vi "Sensor Mesurament from phone and hercules.vi"() -> ()   [LabVIEW 2012]
uses:
  <vilib>/Instr/_visa.llb/VISA Configure Serial Port (Instr).vi
  <vilib>/Utility/file.llb/Write To Spreadsheet File (DBL).vi
  <vilib>/Utility/file.llb/Read From Spreadsheet File (DBL).vi
  <vilib>/Utility/file.llb/Write To Spreadsheet File (string).vi
  <vilib>/Utility/file.llb/Read From Spreadsheet File (string).vi
  <vilib>/Analysis/NI_AALBase.lvlib
panel:
  out "Control Option":string
  out "Dati":dbl[][](array[numeric])
  in  "Tab Control":T1(tab)
  out "?":bool
  in  "QUIT":bool
  out "Off/On":bool
  in  "Unit":u32(ring)=1000 items=["hr"=3600000, "min"=60000, "sec"=1000, "ms"=1]
  in  "Timer":bool
  in  "Magnitude":bool
  in  "Filter":u16
  in  "?":bool
  in  "?":bool
  in  "?":bool
  in  "?":bool
  in  "?":bool
  in  "?":bool
  in  "?":bool
  in  "?":bool
  in  "?":bool
  in  "?":bool
  in  "?":bool
  in  "?":bool
  in  "?":bool
  in  "?":bool
  in  "read bluetooth":bool
  in  "VISA resource name":refnum<visa-resource-name>="COM4"
  out "Bytes at Port":u32
  in  "baud rate (9600)":u32=9600
  in  "stop and Save":bool
  out "dati ist":dbl[](array[numeric])
  out "?":waveform(dbl)[](graph)
  in  "dt":dbl=100.0
  in  "Save path":path=path "C:/Users/leona/Desktop/progetto misure/File/Saves"
  out "start data/time":string
  out "stop data/time":string
  out "Max":dbl[](array[numeric])
  out "Min":dbl[](array[numeric])
  out "Mean":dbl[](array[numeric])
  out "St. dev":dbl[](array[numeric])
  out "Variance":dbl[](array[numeric])
  in  "data bits (8)":u16=8 min=5 max=8 step=1
  in  "parity (0:none)":enum16{"None", "Odd", "Even", "Mark", "Space"}(ring)
  in  "stop bits (10: 1 bit)":u16(ring)=10 items=["1.0"=10, "1.5"=15, "2.0"=20]
  in  "flow control (0:none)":u16(ring) items=["None", "XON/XOFF", "RTS/CTS", "XON/XOFF & RTS/CTS", "DTR/DSR", "XON/XOFF & DTR/DSR"]
  out "Tick count":u32
  in  "Timer":dbl
  in  "Both":bool
  in  "?":bool
  in  "?":bool
  in  "?":bool
  in  "?":bool
  in  "?":bool
  in  "?":bool
  in  "?":bool
  in  "?":bool
  in  "?":bool
  in  "?":bool
  in  "?":bool
  in  "?":bool
  in  "?":bool
  in  "?":bool
  in  "file 1":path
  out "Max 1":dbl[](array[numeric])
  out "Min 1":dbl[](array[numeric])
  out "Mean 1":dbl[](array[numeric])
  out "St. Dev 1":dbl[](array[numeric])
  out "Varian 1":dbl[](array[numeric])
  in  "dt 1":dbl=100.0
  in  "Filter 1":u16
  out "?":waveform(dbl)[](graph)
  out "Varian 2":dbl[](array[numeric])
  out "St. Dev 2":dbl[](array[numeric])
  out "Mean 2":dbl[](array[numeric])
  out "Min 2":dbl[](array[numeric])
  out "Max 2":dbl[](array[numeric])
  in  "file 2":path
  in  "Filter 2":u16
  in  "dt 2":dbl=100.0
  out "Start data 2":string
  out "Stop data 2":string
  out "Start data 1":string
  out "Stop data 1":string
  out "?":waveform(dbl)[](graph)
  in  "Stop Load":bool
  in  "Load":bool
  in  "Filter both":u16
  in  "dt both":dbl=100.0
  out "Dati 1":dbl[][](array[numeric])
  out "Dati 2":dbl[][](array[numeric])
  out "Delta T 1(s)":dbl
  out "Delta T2 (s)":dbl
  in  "?":bool
  in  "?":bool
  in  "?":bool
  in  "?":bool
  in  "?":bool
  in  "?":bool
  in  "?":bool
  in  "?":bool
  in  "?":bool
  in  "?":bool
  in  "?":bool
  in  "?":bool
  in  "?":bool
  in  "?":bool
  out "Waveform Graph":waveform(dbl)[](graph)
  out "?":dbl[][](array[numeric])
  in  "file path":path=path "C:/Users/leona/Desktop/progetto misure/Telefono_COM4/Dati_Telefono_deltaT.log"
  in  "Read file":bool
  out "Max 3":dbl[](array[numeric])
  out "Min 3":dbl[](array[numeric])
  out "Mean 3":dbl[](array[numeric])
  out "St. dev 3":dbl[](array[numeric])
  out "Variance 3":dbl[](array[numeric])
  in  "stop":bool
  in  "Filter 3":u16
  in  "dt 3":dbl=100.0
  out "Stato DIst (disabilitato)":bool
  in  "Lock Distance":bool
  out "Load File":bool
  out "Read Bluetooth":bool
  out "Read File":bool
  out "Admin":bool
  out "Stato locat (disabilitato)":bool
  in  "Lock Location":bool
  in  "Add":bool
  in  "PASS":string
  in  "ID":string
  in  "Show":bool
  out "Username & Password":string[][](array[string])
  in  "Delete":bool
  in  "Delete ID":string
  out "Result":string
  # "You have successfully logged in!"
  # "Read Bluetooth: read data from your phone sensors"
  # "Load file: Let you load old file"
  # "Read File: read data from Hercules software"
  # "Admin option: Admin exclusive options"
  # "xxxxxxxxxxxxxxxxxxxxxxxxxxxxxxxxxxxxx\n\n                       Sensor Project\n\nxxxxxxxxxxxxxxxxxxxxxxxxxxxxxxxxxxxxx"
  # "Acc X"
  # "Acc Y"
  # "Acc Z"
  # "Velo X"
  # "Velo Y"
  # "Velo Z"
  # "Azimuth"
  # "Pitch"
  # "Roll"
  # "Distance"
  # "Lat"
  # "Lon"
  # "Altitude"
  # "Speed"
  # "Connection option"
  # "Timer option"
  # "off/on"
  # "Acc X"
  # "Acc Y"
  # "Acc Z"
  # "Velo X"
  # "Velo Y"
  # "Velo Z"
  # "Azimuth"
  # "Pitch"
  # "Roll"
  # "Distance"
  # "Lat"
  # "Lon"
  # "Altitude"
  # "Speed"
  # "Acc X"
  # "Acc Y"
  # "Acc Z"
  # "Velo X"
  # "Velo Y"
  # "Velo Z"
  # "Azimuth"
  # "Pitch"
  # "Roll"
  # "Distance"
  # "Lat"
  # "Lon"
  # "Altitude"
  # "Speed"
  # "Login option"
  # "Lock option"
  # "Active functions"
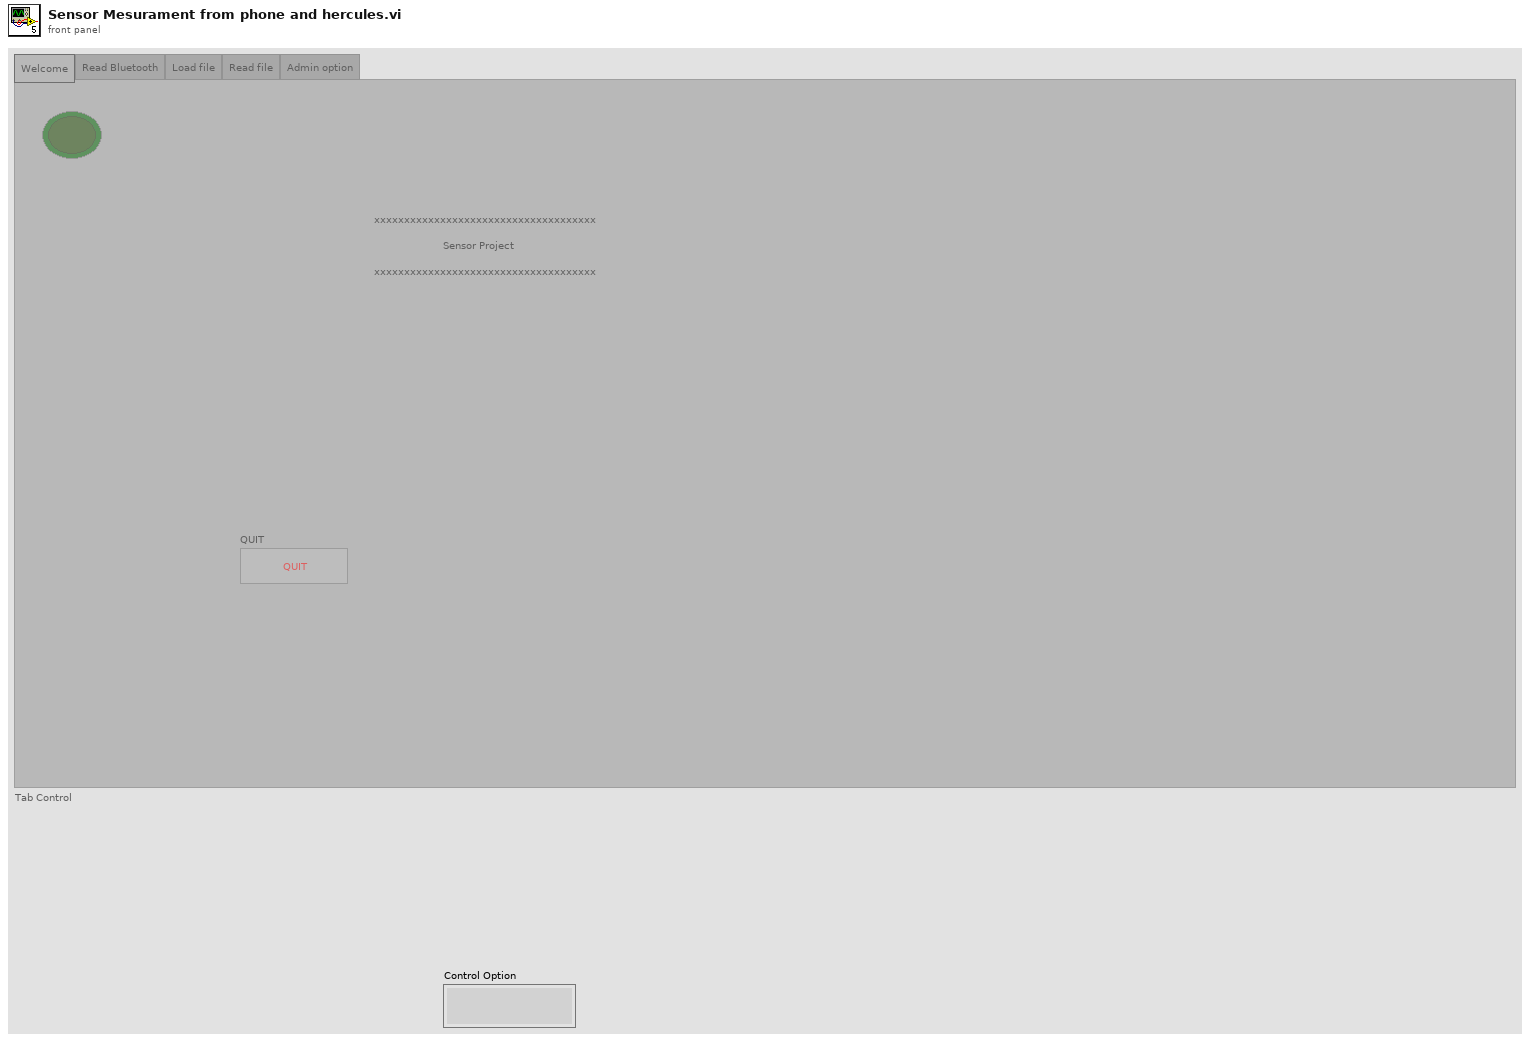
[diagram p1: front panel]
types:
  T1 = enum32{"Welcome", "Read Bluetooth", "Load file", "Read file", "Admin option"}
  T2 = enum8{"Enabled", "Disabled", "Disabled and Grayed Out"}
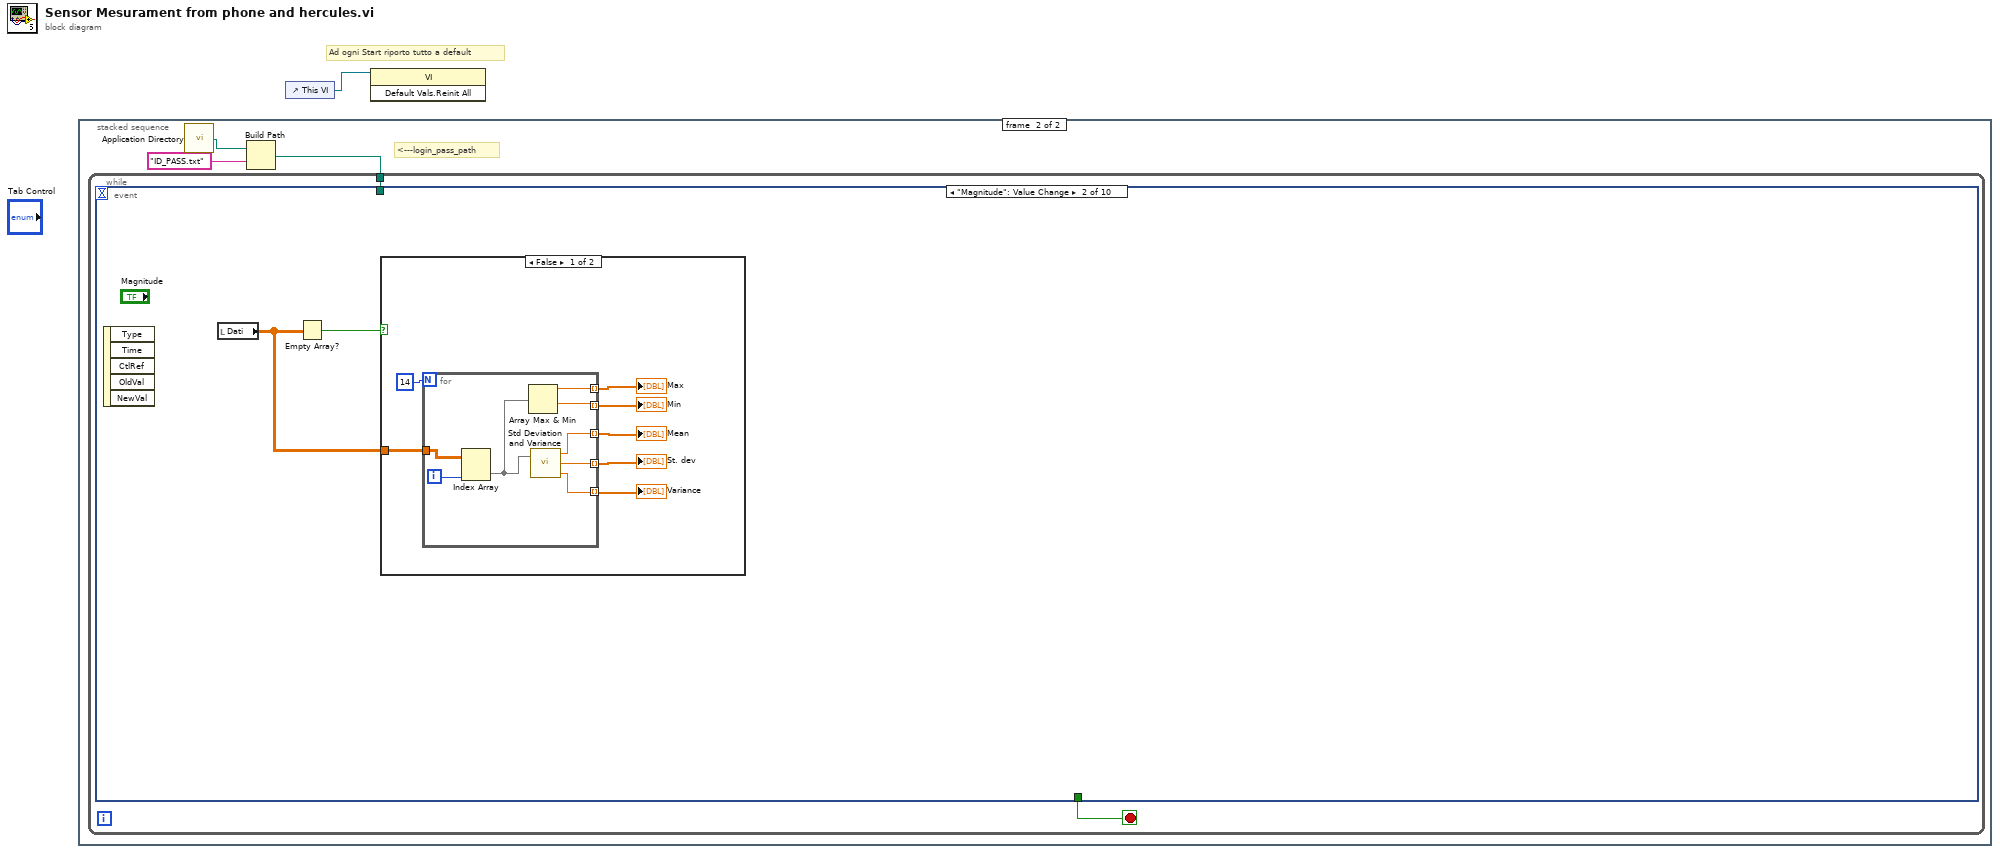
[diagram p0: block diagram]
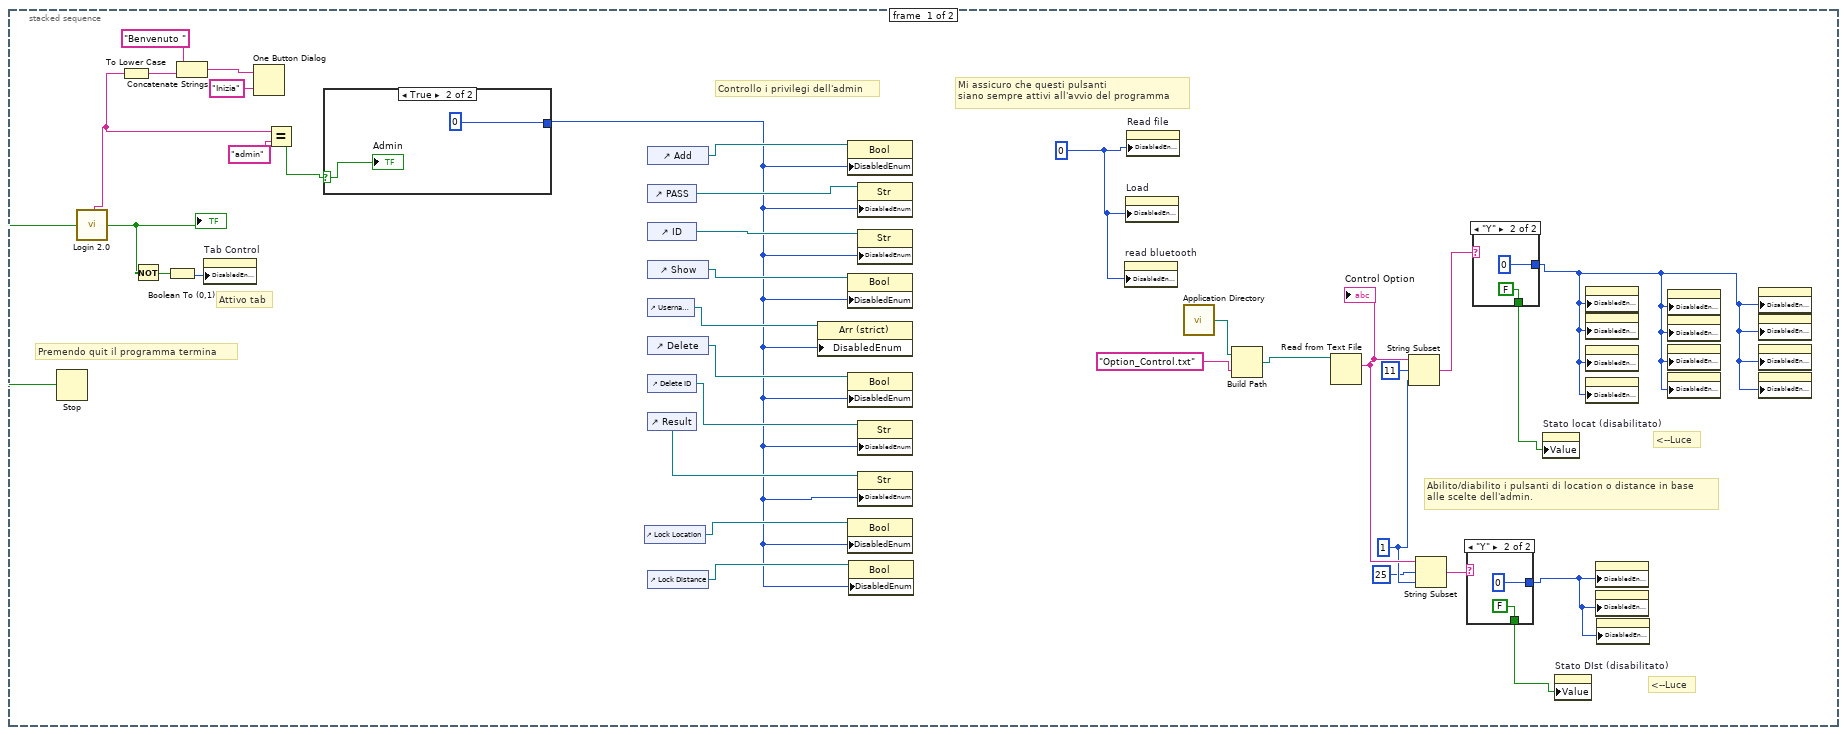
[diagram p2: hidden frame]
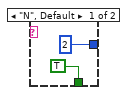
[diagram p3: hidden frame]
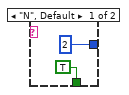
[diagram p4: hidden frame]
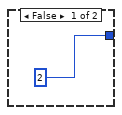
[diagram p5: hidden frame]
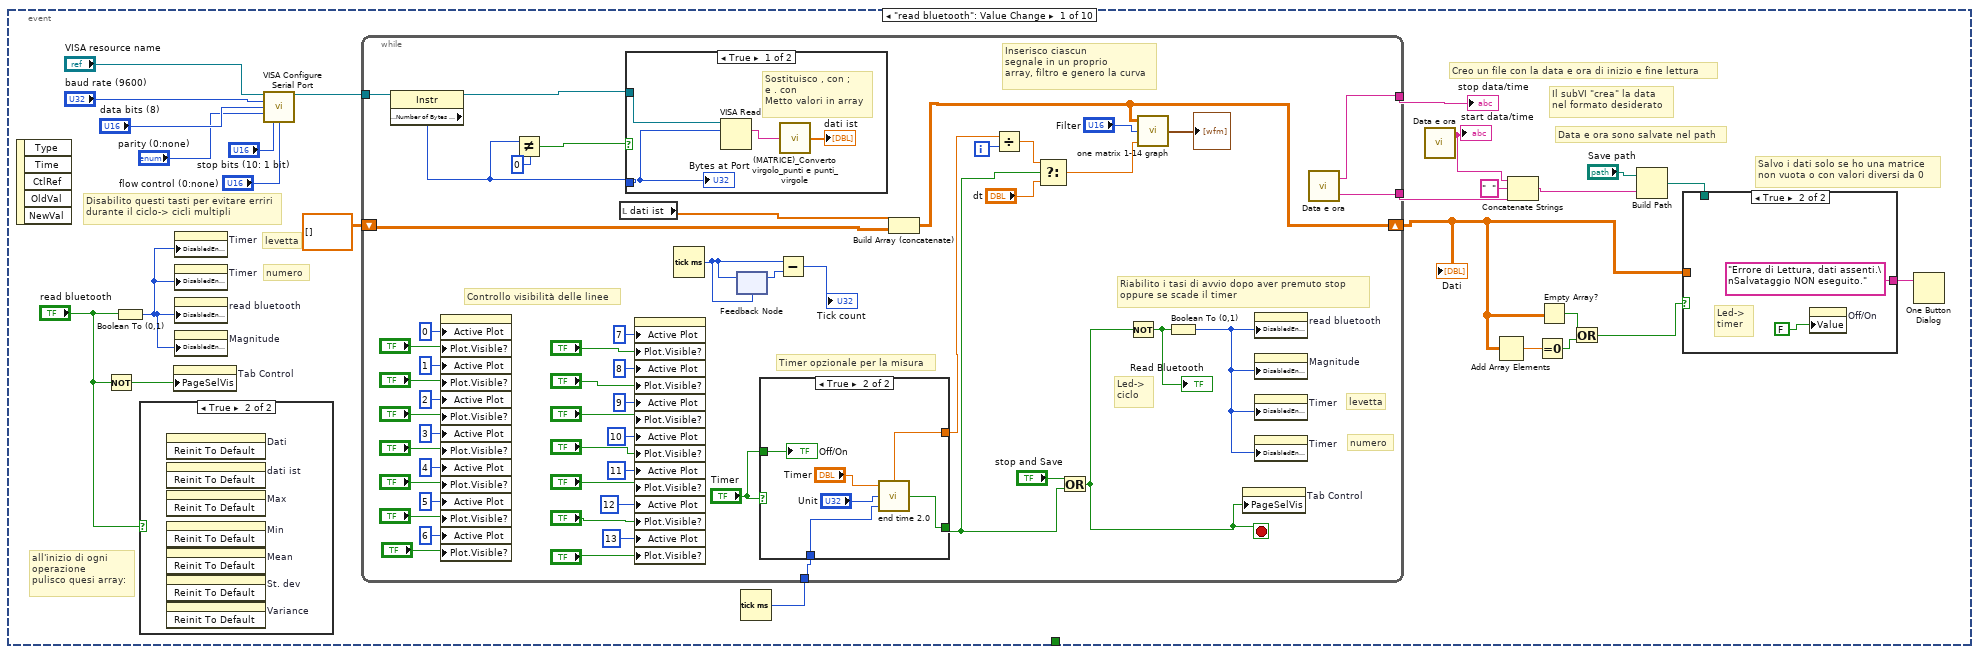
[diagram p6: hidden frame]
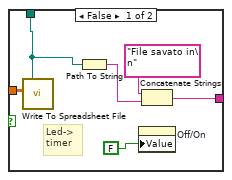
[diagram p8: hidden frame]
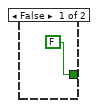
[diagram p9: hidden frame]
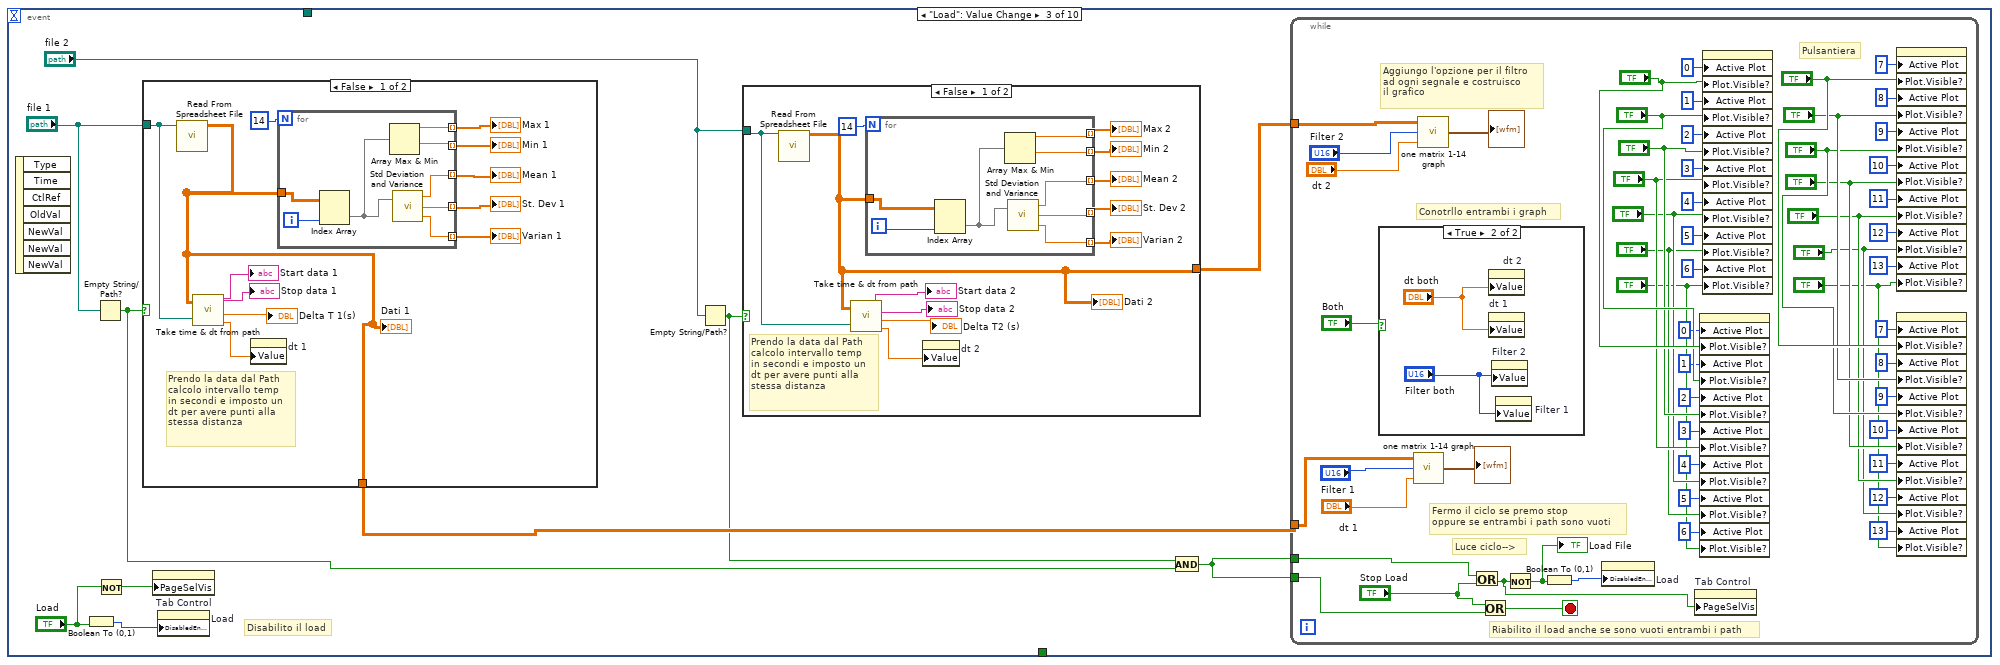
[diagram p12: hidden frame]
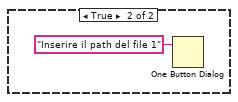
[diagram p14: hidden frame]
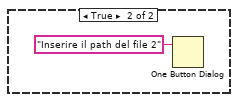
[diagram p15: hidden frame]
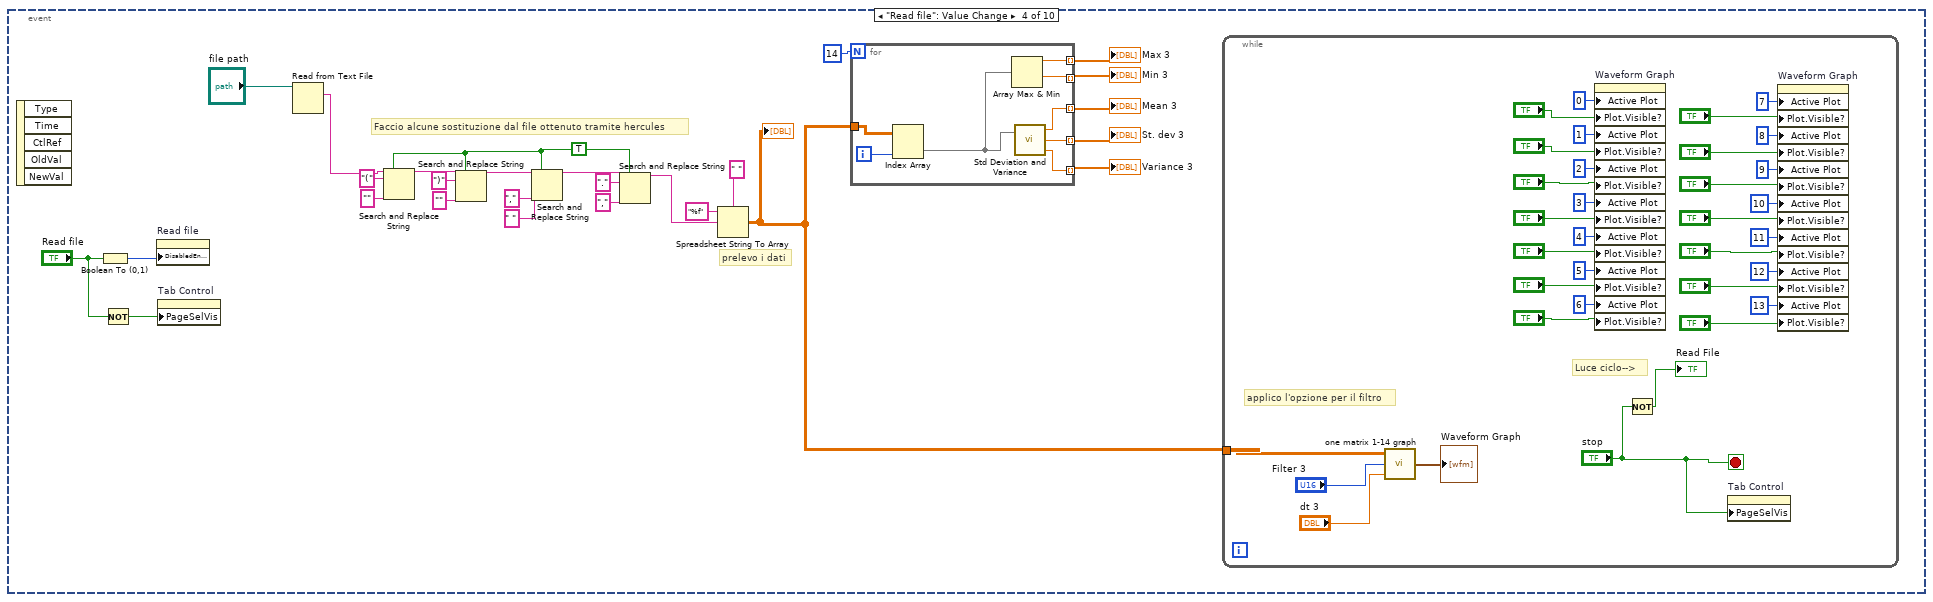
[diagram p16: hidden frame]
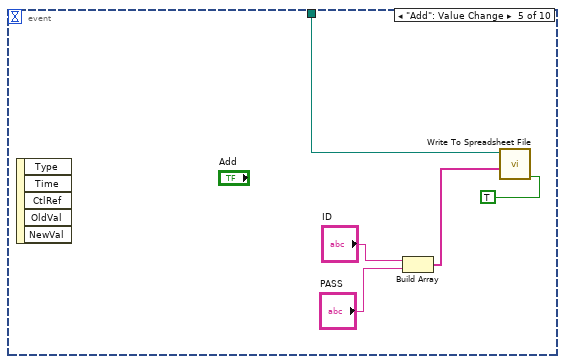
[diagram p17: hidden frame]
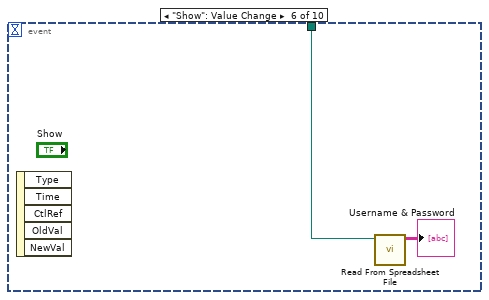
[diagram p18: hidden frame]
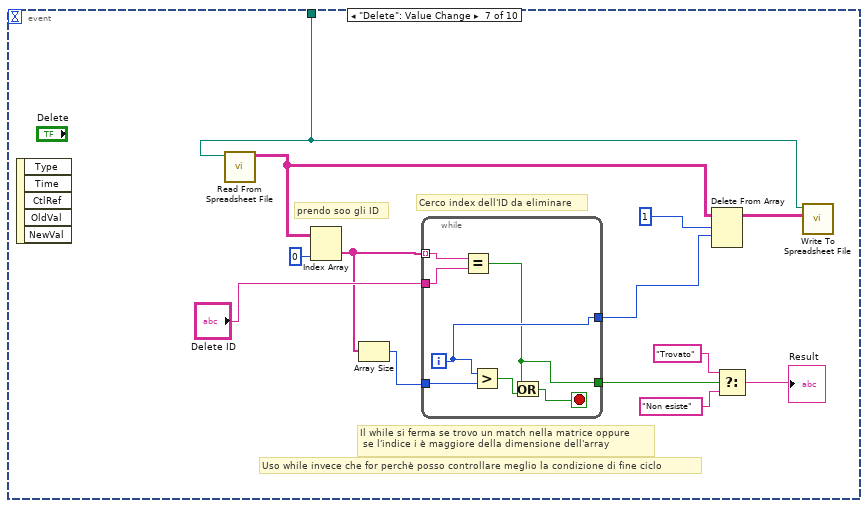
[diagram p19: hidden frame]
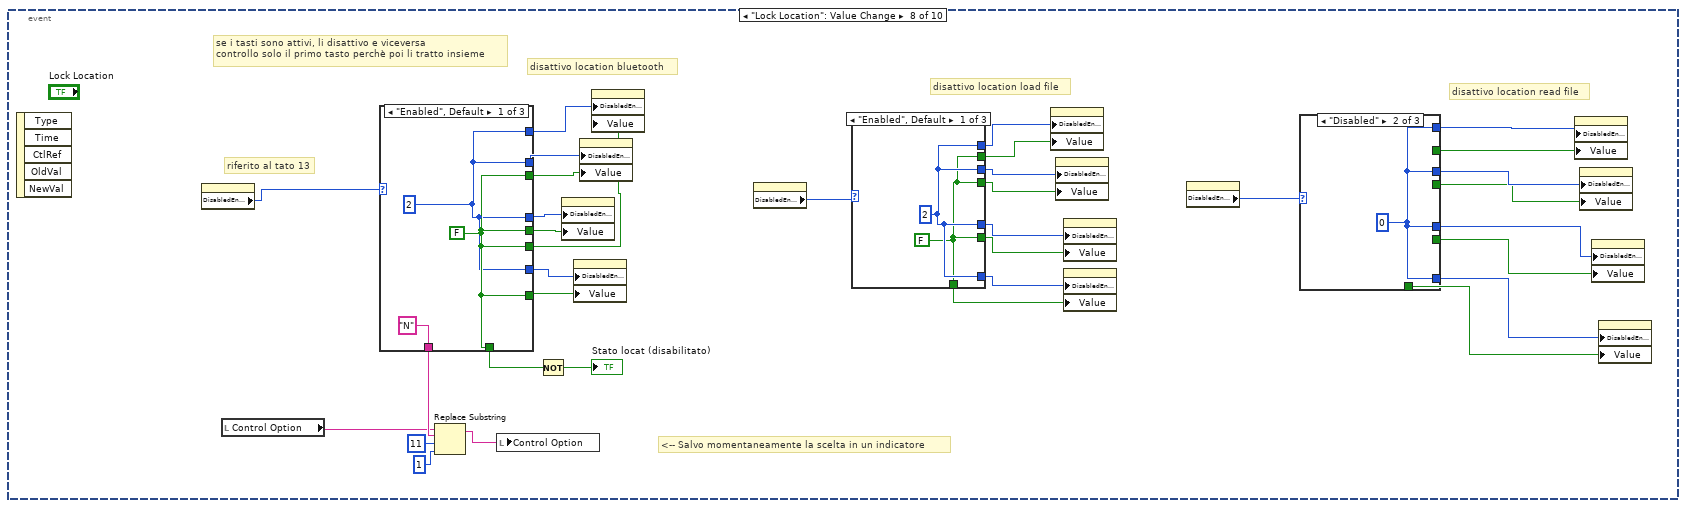
[diagram p20: hidden frame]
diagram:
  # "Ad ogni Start riporto tutto a default"
  n1 = stacked-sequence {
    frame #0 {
      w12 = 1 ("length (rest)")
      w28 = 0
      # "<--Luce"
      # "<--Luce"
      # "Abilito/diabilito i pulsanti di location o distance in base\nalle scelte dell'admin."
      # "Premendo quit il programma termina"
      # "Attivo tab"
      # "Controllo i privilegi dell'admin"
      # "Mi assicuro che questi pulsanti\nsiano sempre attivi all'avvio del programma"
      n2 = call "Login 2.0.vi"() -> ("quit led"=w15:bool, "UTENTE"=w17:string, 2:w16:bool)
      "?" <- w16
      n3 = Stop(stop? (T)=w15) -> ()
      n4 = To Lower Case(string=w17) -> (all lower case string=w21:string)
      n5 = Not(x=w16) -> (.not. x?=w18:bool)
      n6 = Boolean To (0,1)(Boolean=w18) -> (0, 1=w27:i16)
      n7 = Concatenate Strings("Benvenuto " ("string"), w21) -> (w23:string)
      n8 = property on="Tab Control" class="TabCtl (strict)"("DisabledEnum"=w27) -> ()  [unwired: 2 in, 2 out]
      n9 = One Button Dialog(message=w23, button name ("OK")="Inizia") -> ()  [unwired: 1 out]
      n10 = Equal?(x=w17, y="admin") -> (x = y?=w26:bool)
      n11 = case shown="True" w26 {
        selector: w26 -> [_ w47]
        tunnel: [2 0] -> w19
        frame False {
        }
        frame True {
          "Admin" <- w47
        }
      }
      n12 = control-ref of="Lock Location"() -> (w25:refnum<vi>)
      n13 = control-ref of="Add"() -> (w36:refnum<vi>)
      n14 = control-ref of="PASS"() -> (w35:refnum<vi>)
      n15 = control-ref of="ID"() -> (w34:refnum<vi>)
      n16 = control-ref of="Show"() -> (w33:refnum<vi>)
      n17 = control-ref of="Username & Password"() -> (w32:refnum<vi>)
      n18 = control-ref of="Delete"() -> (w31:refnum<vi>)
      n19 = control-ref of="Delete ID"() -> (w30:refnum<vi>)
      n20 = control-ref of="Result"() -> (w29:refnum<vi>)
      n21 = control-ref of="Lock Distance"() -> (w20:refnum<vi>)
      n22 = property class="Arr (strict)"(reference=w32, "DisabledEnum"=w19) -> ()  [unwired: 1 in, 2 out]
      n23 = property class="Bool"(reference=w36, "DisabledEnum"=w19) -> ()  [unwired: 1 in, 2 out]
      n24 = property class="Bool"(reference=w33, "DisabledEnum"=w19) -> ()  [unwired: 1 in, 2 out]
      n25 = property class="Bool"(reference=w31, "DisabledEnum"=w19) -> ()  [unwired: 1 in, 2 out]
      n26 = property class="Bool"(reference=w25, "DisabledEnum"=w19) -> ()  [unwired: 1 in, 2 out]
      n27 = property class="Bool"(reference=w20, "DisabledEnum"=w19) -> ()  [unwired: 1 in, 2 out]
      n28 = property class="Str"(reference=w35, "DisabledEnum"=w19) -> ()  [unwired: 1 in, 2 out]
      n29 = property class="Str"(reference=w34, "DisabledEnum"=w19) -> ()  [unwired: 1 in, 2 out]
      n30 = property class="Str"(reference=w30, "DisabledEnum"=w19) -> ()  [unwired: 1 in, 2 out]
      n31 = property class="Str"(reference=w29, "DisabledEnum"=w19) -> ()  [unwired: 1 in, 2 out]
      n32 = property on="read bluetooth" class="Bool"("DisabledEnum"=w28) -> ()  [unwired: 2 in, 2 out]
      n33 = property on="Load" class="Bool"("DisabledEnum"=w28) -> ()  [unwired: 2 in, 2 out]
      n34 = property on="Read file" class="Bool"("DisabledEnum"=w28) -> ()  [unwired: 2 in, 2 out]
      n35 = call <vilib>:"Application Directory.vi"() -> ("Application Directory"=w4:path)
      n36 = Build Path(base path=w4, name or relative path="Option_Control.txt") -> (appended path=w2:path)
      n37 = Read from Text File(file (use dialog)=w2) -> (text=w13:string)  [unwired: 3 in, 3 out]
      "Control Option" <- w13
      n38 = String Subset(string=w13, offset (0)=11, length (rest)=w12) -> (substring=w10:string)
      n39 = String Subset(string=w13, offset (0)=25, length (rest)=w12) -> (substring=w8:string)
      n40 = case shown="\"Y\"" w8 {
        tunnel: [2 0] -> w7
        tunnel: [TRUE FALSE] -> w5
        frame "N", Default {
        }
        frame "Y" {
        }
      }
      n41 = case shown="\"Y\"" w10 {
        tunnel: [2 0] -> w9
        tunnel: [TRUE FALSE] -> w6
        frame "N", Default {
        }
        frame "Y" {
        }
      }
      n42 = property on="Stato locat (disabilitato)" class="Bool (strict)"("Value"=w6) -> ()  [unwired: 2 in, 2 out]
      n43 = property on="Stato DIst (disabilitato)" class="Bool (strict)"("Value"=w5) -> ()  [unwired: 2 in, 2 out]
      n44 = property class="Bool (strict)"("DisabledEnum"=w9) -> ()  [unwired: 2 in, 2 out]
      n45 = property class="Bool (strict)"("DisabledEnum"=w9) -> ()  [unwired: 2 in, 2 out]
      n46 = property class="Bool (strict)"("DisabledEnum"=w9) -> ()  [unwired: 2 in, 2 out]
      n47 = property class="Bool (strict)"("DisabledEnum"=w9) -> ()  [unwired: 2 in, 2 out]
      n48 = property class="Bool (strict)"("DisabledEnum"=w7) -> ()  [unwired: 2 in, 2 out]
      n49 = property class="Bool (strict)"("DisabledEnum"=w7) -> ()  [unwired: 2 in, 2 out]
      n50 = property class="Bool (strict)"("DisabledEnum"=w7) -> ()  [unwired: 2 in, 2 out]
      n51 = property class="Bool (strict)"("DisabledEnum"=w9) -> ()  [unwired: 2 in, 2 out]
      n52 = property class="Bool (strict)"("DisabledEnum"=w9) -> ()  [unwired: 2 in, 2 out]
      n53 = property class="Bool (strict)"("DisabledEnum"=w9) -> ()  [unwired: 2 in, 2 out]
      n54 = property class="Bool (strict)"("DisabledEnum"=w9) -> ()  [unwired: 2 in, 2 out]
      n55 = property class="Bool (strict)"("DisabledEnum"=w9) -> ()  [unwired: 2 in, 2 out]
      n56 = property class="Bool (strict)"("DisabledEnum"=w9) -> ()  [unwired: 2 in, 2 out]
      n57 = property class="Bool (strict)"("DisabledEnum"=w9) -> ()  [unwired: 2 in, 2 out]
      n58 = property class="Bool (strict)"("DisabledEnum"=w9) -> ()  [unwired: 2 in, 2 out]
    }
    frame #1 {
      # "<---login_pass_path"
      n59 = call <vilib>:"Application Directory.vi"() -> ("Application Directory"=w51:path)
      n60 = Build Path(base path=w51, name or relative path="ID_PASS.txt") -> (appended path=w49:path)
      n61 = while {
        tunnel: w49 -> [w53]
        stop <- w52 stop-if-true
        n62 = event shown="[1] \"Magnitude\": Value Change" {
          selector: _ -> [_ _ _ _ _ _ _ _ _ _]
          dyn-events: _ -> [_ _ _ _ _ _ _ _ _ _]
          timeout: _ -> [_ _ _ _ _ _ _ _ _ _]
          tunnel: w53 -> [_ _ _ _ w351 w356 w358 _ _ _]
          tunnel: [_ _ _ _ _ _ _ _ _ "QUIT"] -> w52
          event "read bluetooth": Value Change {
            # "numero"
            # "levetta"
            # "all'inizio di ogni \noperazione\npulisco quesi array:"
            # "Salvo i dati solo se ho una matrice\nnon vuota o con valori diversi da 0"
            # "Disabilito questi tasti per evitare erriri\ndurante il ciclo-> cicli multipli"
            # "Data e ora sono salvate nel path"
            # "Il subVI \"crea\" la data\nnel formato desiderato"
            # "Creo un file con la data e ora di inizio e fine lettura"
            n63 = event-data() -> ()  [unwired: 1 in, 5 out]
            n64 = Not(x="read bluetooth") -> (.not. x?=w57:bool)
            n65 = Boolean To (0,1)(Boolean="read bluetooth") -> (0, 1=w55:i16)
            n66 = case shown="True" "read bluetooth" {
              frame False {
              }
              frame True {
                n67 = invoke on="Dati" class="Arr (strict)" method="Reinit To Default"() -> ()  [unwired: 3 in, 3 out]
                n68 = invoke on="dati ist" class="Arr (strict)" method="Reinit To Default"() -> ()  [unwired: 3 in, 3 out]
                n69 = invoke on="Max" class="Arr (strict)" method="Reinit To Default"() -> ()  [unwired: 3 in, 3 out]
                n70 = invoke on="Min" class="Arr (strict)" method="Reinit To Default"() -> ()  [unwired: 3 in, 3 out]
                n71 = invoke on="Mean" class="Arr (strict)" method="Reinit To Default"() -> ()  [unwired: 3 in, 3 out]
                n72 = invoke on="St. dev" class="Arr (strict)" method="Reinit To Default"() -> ()  [unwired: 3 in, 3 out]
                n73 = invoke on="Variance" class="Arr (strict)" method="Reinit To Default"() -> ()  [unwired: 3 in, 3 out]
              }
            }
            n74 = property on="Tab Control" class="TabCtl (strict)"("PageSelVis"=w57) -> ()  [unwired: 2 in, 2 out]
            n75 = property on="Timer" class="DigNum (strict)"("DisabledEnum"=w55) -> ()  [unwired: 2 in, 2 out]
            n76 = property on="Timer" class="Bool (strict)"("DisabledEnum"=w55) -> ()  [unwired: 2 in, 2 out]
            n77 = property on="read bluetooth" class="Bool"("DisabledEnum"=w55) -> ()  [unwired: 2 in, 2 out]
            n78 = property on="Magnitude" class="Bool"("DisabledEnum"=w55) -> ()  [unwired: 2 in, 2 out]
            n79 = call-poly "VISA Configure Serial Port"("VISA resource name"="VISA resource name", "baud rate (9600)"="baud rate (9600)", "data bits (8)"="data bits (8)", "parity (0:none)"="parity (0:none)", "stop bits (10: 1 bit)"="stop bits (10: 1 bit)", "flow control (0:none)"="flow control (0:none)") -> ("VISA resource name out"=w78:refnum<visa-resource-name>)  [unwired: 8 in, 1 out]
            n80 = Tick Count (ms)() -> (millisecond timer value=w54:u32)
            n81 = while {
              tunnel: w78 -> [w141]
              shift-right: [w87] -> w58
              shift-left: dbl[][] [] -> [w135]
              tunnel: [w111] -> w73
              tunnel: [w110] -> w74
              tunnel: w54 -> [w102]
              i -> [w89]
              stop <- w98 stop-if-true
              # "numero"
              # "levetta"
              # "Timer opzionale per la misura"
              # "Led-> \nciclo"
              # "Riabilito i tasi di avvio dopo aver premuto stop \noppure se scade il timer"
              # "Inserisco ciascun\nsegnale in un proprio\narray, filtro e genero la curva"
              # "Controllo visibilità delle linee"
              n82 = property class="Instr"(reference=w141) -> (reference out=w140:refnum<visa-resource-name>, "Serial Settings:Number of Bytes at Serial Port"=w137:u32)  [unwired: 1 in, 1 out]
              n83 = property class="WFGraph (strict)"("Active Plot"=u32 0, "Plot.Visible?"="?", "Active Plot"=u32 1, "Plot.Visible?"="?", "Active Plot"=u32 2, "Plot.Visible?"="?", "Active Plot"=u32 3, "Plot.Visible?"="?", "Active Plot"=u32 4, "Plot.Visible?"="?", "Active Plot"=u32 5, "Plot.Visible?"="?", "Active Plot"=u32 6, "Plot.Visible?"="?") -> ()  [unwired: 2 in, 2 out]
              n84 = Not Equal?(x=w137, y=u32 0 ("x")) -> (x != y?=w139:bool)
              n85 = local read "dati ist"() -> (w136:dbl[])
              n86 = case shown="True" w139 {
                tunnel: w137 -> [w152 _]
                tunnel: w140 -> [w151 _]
                frame True {
                  # "Sostituisco , con ;\ne . con \nMetto valori in array"
                  n87 = VISA Read(VISA resource name=w151, byte count=w152) -> (read buffer=w150:string)  [unwired: 1 in, 3 out]
                  n88 = call "(MATRICE)_Converto virgolo_punti e punti_virgole.vi"("Stringa Input"=w150) -> ("appended array"=→"dati ist":dbl[])
                  "Bytes at Port" <- w152
                }
                frame False {
                }
              }
              n89 = property class="WFGraph (strict)"("Active Plot"=u32 7, "Plot.Visible?"="?", "Active Plot"=u32 8, "Plot.Visible?"="?", "Active Plot"=u32 9, "Plot.Visible?"="?", "Active Plot"=u32 10, "Plot.Visible?"="?", "Active Plot"=u32 11, "Plot.Visible?"="?", "Active Plot"=u32 12, "Plot.Visible?"="?", "Active Plot"=u32 13, "Plot.Visible?"="?") -> ()  [unwired: 2 in, 2 out]
              n90 = Tick Count (ms)() -> (millisecond timer value=w96:u32)
              n91 = feedback #1(w96) -> (w103:u32)
              n92 = feedback-in #1(w96) -> ()
              n93 = case shown="True" "Timer" {
                tunnel: w102 -> [_ w145]
                tunnel: [FALSE ("Boolean") w144] -> w92
                tunnel: "Timer" -> [_ w148]
                tunnel: [_ w143] -> w90
                frame False {
                }
                frame True {
                  n94 = call "end time 2.0.vi"("start"=w145, "unit"="Unit", "End time"="Timer") -> ("Boolean"=w144:bool, "dt ideale"=w143:dbl)
                  "Off/On" <- w148
                }
              }
              n95 = Subtract(x=w96, y=w103) -> (x-y=→"Tick count":u32)
              n96 = Build Array (concatenate)(w136, w135) -> (w87:dbl[][])
              n97 = Divide(x=w90, y=w89) -> (x/y=w91:dbl)
              n98 = Select(t=w91, s=w92, f="dt") -> (s? t:f=w88:dbl)
              n99 = Or(x="stop and Save", y=w92) -> (x .or. y?=w98:bool)
              n100 = Not(x=w98) -> (.not. x?=w100:bool)
              "Read Bluetooth" <- w100
              n101 = call "one matrix 1-14 graph.vi"("dt"=w88, "Applica filtro 4"="Filter", "Dati 2"=w87) -> ("Waveform Graph"=→"?":waveform(dbl)[])
              n102 = Boolean To (0,1)(Boolean=w100) -> (0, 1=w97:i16)
              n103 = property on="Tab Control" class="TabCtl (strict)"("PageSelVis"=w98) -> ()  [unwired: 2 in, 2 out]
              n104 = property on="read bluetooth" class="Bool"("DisabledEnum"=w97) -> ()  [unwired: 2 in, 2 out]
              n105 = property on="Magnitude" class="Bool"("DisabledEnum"=w97) -> ()  [unwired: 2 in, 2 out]
              n106 = property on="Timer" class="Bool (strict)"("DisabledEnum"=w97) -> ()  [unwired: 2 in, 2 out]
              n107 = property on="Timer" class="DigNum (strict)"("DisabledEnum"=w97) -> ()  [unwired: 2 in, 2 out]
              n108 = call "Data e ora.vi"() -> ("Data_ora_txt"=w111:string, "date_ora"=w110:string)
            }
            "stop data/time" <- w74
            "Dati" <- w58
            n109 = call "Data e ora.vi"() -> ("date_ora"=w70:string)  [unwired: 1 out]
            "start data/time" <- w70
            n110 = Add Array Elements(numeric array=w58) -> (sum=w60:dbl)
            n111 = Concatenate Strings(w70, "  " ("string"), w73) -> (w71:string)
            n112 = Equal To 0?(x=w60) -> (x = 0?=w61:bool)
            n113 = Empty Array?(array=w58) -> (empty?=w62:bool)
            n114 = Or(x=w62, y=w61) -> (x .or. y?=w59:bool)
            n115 = Build Path(base path="Save path", name or relative path=w71) -> (appended path=w69:path)
            n116 = case shown="True" w59 {
              tunnel: w69 -> [w84 _]
              tunnel: [w81 "Errore di Lettura, dati assenti.\nSalvataggio NON eseguito."] -> w68
              tunnel: w58 -> [w80 _]
              frame False {
                # "Led-> \ntimer"
                n117 = call-poly <vilib>:"Write To Spreadsheet File.vi"("2D data"=w80, "file path (dialog if empty)"=w84) -> ()  [unwired: 6 in, 1 out]
                n118 = Path To String(path=w84) -> (string=w83:string)
                n119 = property on="Off/On" class="Bool (strict)"("Value"=FALSE) -> ()  [unwired: 2 in, 2 out]
                n120 = Concatenate Strings("File savato in\n" ("string"), w83) -> (w81:string)
              }
              frame True {
                # "Led-> \ntimer"
                n121 = property on="Off/On" class="Bool (strict)"("Value"=FALSE) -> ()  [unwired: 2 in, 2 out]
              }
            }
            n122 = One Button Dialog(message=w68) -> ()  [unwired: 1 in, 1 out]
          }
          event "Magnitude": Value Change {
            n123 = event-data() -> ()  [unwired: 1 in, 5 out]
            n124 = local read "Dati"() -> (w153:dbl[][])
            n125 = Empty Array?(array=w153) -> (empty?=w154:bool)
            n126 = case shown="False" w154 {
              tunnel: w153 -> [w160 _]
              frame False {
                n127 = for {
                  N: 14 -> [_]
                  tunnel: w160 -> [w169]
                  tunnel: [w167] -> w157 mode=indexing
                  tunnel: [w166] -> w156 mode=indexing
                  tunnel: [w165] -> w155 mode=indexing
                  tunnel: [w163] -> w159 mode=indexing
                  tunnel: [w162] -> w158 mode=indexing
                  i -> [w168]
                  n128 = Index Array(array=w169, index (col)=w168) -> (element=w164:dbl[])  [unwired: 1 in]
                  n129 = Array Max & Min(array=w164) -> (max value=w163:dbl, min value=w162:dbl)  [unwired: 2 out]
                  n130 = call <vilib>:"Std Deviation and Variance.vi"("X"=w164) -> ("mean"=w167:dbl, "standard deviation"=w166:dbl, "variance"=w165:dbl)  [unwired: 1 in]
                }
                "Max" <- w159
                "Min" <- w158
                "Mean" <- w157
                "St. dev" <- w156
                "Variance" <- w155
              }
              frame True {
              }
            }
          }
          event "Load": Value Change {
            # "Disabilito il load"
            n131 = event-data() -> ()  [unwired: 1 in, 7 out]
            n132 = Boolean To (0,1)(Boolean="Load") -> (0, 1=w172:i16)
            n133 = Empty String/Path?(string/path="file 1") -> (empty?=w175:bool)
            n134 = Not(x="Load") -> (.not. x?=w170:bool)
            n135 = case shown="False" w175 {
              tunnel: "file 1" -> [w245 _]
              tunnel: [w244 _] -> w179
              frame False {
                # "Prendo la data dal Path\ncalcolo intervallo temp\nin secondi e imposto un\ndt per avere punti alla \nstessa distanza"
                n136 = call-poly <vilib>:"Read From Spreadsheet File.vi"("file path (dialog if empty)"=w245) -> ("all rows"=w244:dbl[][])  [unwired: 6 in, 4 out]
                "Dati 1" <- w244
                n137 = call "Take time & dt from path.vi"("Array"=w244, "path"=w245) -> ("Start data 1"=→"Start data 1":string, "Stop data 1"=→"Stop data 1":string, "Delta T (s)"=→"Delta T 1(s)":dbl, "dt id (ms)"=w240:dbl)
                n138 = property on="dt 1" class="DigNum (strict)"("Value"=w240) -> ()  [unwired: 2 in, 2 out]
                n139 = for {
                  N: 14 -> [_]
                  tunnel: w244 -> [w259]
                  tunnel: [w257] -> w248 mode=indexing
                  tunnel: [w256] -> w247 mode=indexing
                  tunnel: [w255] -> w246 mode=indexing
                  tunnel: [w254] -> w250 mode=indexing
                  tunnel: [w253] -> w249 mode=indexing
                  i -> [w258]
                  n140 = Index Array(array=w259, index (col)=w258) -> (element=w252:dbl[])  [unwired: 1 in]
                  n141 = Array Max & Min(array=w252) -> (max value=w254:dbl, min value=w253:dbl)  [unwired: 2 out]
                  n142 = call <vilib>:"Std Deviation and Variance.vi"("X"=w252) -> ("mean"=w257:dbl, "standard deviation"=w256:dbl, "variance"=w255:dbl)  [unwired: 1 in]
                }
                "Max 1" <- w250
                "Min 1" <- w249
                "Mean 1" <- w248
                "St. Dev 1" <- w247
                "Varian 1" <- w246
              }
              frame True {
                n143 = One Button Dialog(message="Inserire il path del file 1") -> ()  [unwired: 1 in, 1 out]
              }
            }
            n144 = property on="Tab Control" class="TabCtl (strict)"("PageSelVis"=w170) -> ()  [unwired: 2 in, 2 out]
            n145 = property on="Load" class="Bool"("DisabledEnum"=w172) -> ()  [unwired: 2 in, 2 out]
            n146 = Empty String/Path?(string/path="file 2") -> (empty?=w177:bool)
            n147 = case shown="False" w177 {
              tunnel: "file 2" -> [w266 _]
              tunnel: [w265 _] -> w178
              frame False {
                # "Prendo la data dal Path\ncalcolo intervallo temp\nin secondi e imposto un\ndt per avere punti alla \nstessa distanza"
                n148 = call-poly <vilib>:"Read From Spreadsheet File.vi"("file path (dialog if empty)"=w266) -> ("all rows"=w265:dbl[][])  [unwired: 6 in, 4 out]
                "Dati 2" <- w265
                n149 = call "Take time & dt from path.vi"("Array"=w265, "path"=w266) -> ("Start data 1"=→"Start data 2":string, "Stop data 1"=→"Stop data 2":string, "Delta T (s)"=→"Delta T2 (s)":dbl, "dt id (ms)"=w261:dbl)
                n150 = for {
                  N: 14 -> [_]
                  tunnel: w265 -> [w273]
                  tunnel: [w279] -> w269 mode=indexing
                  tunnel: [w278] -> w268 mode=indexing
                  tunnel: [w277] -> w267 mode=indexing
                  tunnel: [w276] -> w271 mode=indexing
                  tunnel: [w275] -> w270 mode=indexing
                  i -> [w280]
                  n151 = Index Array(array=w273, index (col)=w280) -> (element=w274:dbl[])  [unwired: 1 in]
                  n152 = Array Max & Min(array=w274) -> (max value=w276:dbl, min value=w275:dbl)  [unwired: 2 out]
                  n153 = call <vilib>:"Std Deviation and Variance.vi"("X"=w274) -> ("mean"=w279:dbl, "standard deviation"=w278:dbl, "variance"=w277:dbl)  [unwired: 1 in]
                }
                "Max 2" <- w271
                "Min 2" <- w270
                "Mean 2" <- w269
                "St. Dev 2" <- w268
                "Varian 2" <- w267
                n154 = property on="dt 2" class="DigNum (strict)"("Value"=w261) -> ()  [unwired: 2 in, 2 out]
              }
              frame True {
                n155 = One Button Dialog(message="Inserire il path del file 2") -> ()  [unwired: 1 in, 1 out]
              }
            }
            n156 = And(x=w177, y=w175) -> (x .and. y?=w176:bool)
            n157 = while {
              tunnel: w179 -> [w194]
              tunnel: w178 -> [w195]
              tunnel: w176 -> [w187]
              tunnel: w176 -> [w186]
              stop <- w184 stop-if-true
              # "Luce ciclo-->"
              # "Conotrllo entrambi i graph"
              # "Pulsantiera"
              # "Riabilito il load anche se sono vuoti entrambi i path"
              # "Fermo il ciclo se premo stop \noppure se entrambi i path sono vuoti"
              # "Aggiungo l'opzione per il filtro\nad ogni segnale e costruisco\nil grafico"
              n158 = case shown="True" "Both" {
                frame False {
                }
                frame True {
                  n159 = property on="dt 2" class="DigNum (strict)"("Value"="dt both") -> ()  [unwired: 2 in, 2 out]
                  n160 = property on="dt 1" class="DigNum (strict)"("Value"="dt both") -> ()  [unwired: 2 in, 2 out]
                  n161 = property on="Filter 2" class="DigNum (strict)"("Value"="Filter both") -> ()  [unwired: 2 in, 2 out]
                  n162 = property on="Filter 1" class="DigNum (strict)"("Value"="Filter both") -> ()  [unwired: 2 in, 2 out]
                }
              }
              n163 = call "one matrix 1-14 graph.vi"("dt"="dt 1", "Applica filtro 4"="Filter 1", "Dati 2"=w194) -> ("Waveform Graph"=→"?":waveform(dbl)[])
              n164 = call "one matrix 1-14 graph.vi"("dt"="dt 2", "Applica filtro 4"="Filter 2", "Dati 2"=w195) -> ("Waveform Graph"=→"?":waveform(dbl)[])
              n165 = Or(x=w187, y="Stop Load") -> (x .or. y?=w180:bool)
              n166 = Or(x="Stop Load", y=w186) -> (x .or. y?=w184:bool)
              n167 = Not(x=w180) -> (.not. x?=w181:bool)
              "Load File" <- w181
              n168 = Boolean To (0,1)(Boolean=w181) -> (0, 1=w182:i16)
              n169 = property on="Load" class="Bool"("DisabledEnum"=w182) -> ()  [unwired: 2 in, 2 out]
              n170 = property on="Tab Control" class="TabCtl (strict)"("PageSelVis"=w180) -> ()  [unwired: 2 in, 2 out]
              n171 = property class="WFGraph (strict)"("Active Plot"=u32 0, "Plot.Visible?"="?", "Active Plot"=u32 1, "Plot.Visible?"="?", "Active Plot"=u32 2, "Plot.Visible?"="?", "Active Plot"=u32 3, "Plot.Visible?"="?", "Active Plot"=u32 4, "Plot.Visible?"="?", "Active Plot"=u32 5, "Plot.Visible?"="?", "Active Plot"=u32 6, "Plot.Visible?"="?") -> ()  [unwired: 2 in, 2 out]
              n172 = property class="WFGraph (strict)"("Active Plot"=u32 0, "Plot.Visible?"="?", "Active Plot"=u32 1, "Plot.Visible?"="?", "Active Plot"=u32 2, "Plot.Visible?"="?", "Active Plot"=u32 3, "Plot.Visible?"="?", "Active Plot"=u32 4, "Plot.Visible?"="?", "Active Plot"=u32 5, "Plot.Visible?"="?", "Active Plot"=u32 6, "Plot.Visible?"="?") -> ()  [unwired: 2 in, 2 out]
              n173 = property class="WFGraph (strict)"("Active Plot"=u32 7, "Plot.Visible?"="?", "Active Plot"=u32 8, "Plot.Visible?"="?", "Active Plot"=u32 9, "Plot.Visible?"="?", "Active Plot"=u32 10, "Plot.Visible?"="?", "Active Plot"=u32 11, "Plot.Visible?"="?", "Active Plot"=u32 12, "Plot.Visible?"="?", "Active Plot"=u32 13, "Plot.Visible?"="?") -> ()  [unwired: 2 in, 2 out]
              n174 = property class="WFGraph (strict)"("Active Plot"=u32 7, "Plot.Visible?"="?", "Active Plot"=u32 8, "Plot.Visible?"="?", "Active Plot"=u32 9, "Plot.Visible?"="?", "Active Plot"=u32 10, "Plot.Visible?"="?", "Active Plot"=u32 11, "Plot.Visible?"="?", "Active Plot"=u32 12, "Plot.Visible?"="?", "Active Plot"=u32 13, "Plot.Visible?"="?") -> ()  [unwired: 2 in, 2 out]
            }
          }
          event "Read file": Value Change {
            w293 = TRUE ("replace all? (F)")
            # "prelevo i dati"
            # "Faccio alcune sostituzione dal file ottenuto tramite hercules"
            n175 = event-data() -> ()  [unwired: 1 in, 5 out]
            n176 = Boolean To (0,1)(Boolean="Read file") -> (0, 1=w284:i16)
            n177 = Not(x="Read file") -> (.not. x?=w282:bool)
            n178 = property on="Read file" class="Bool"("DisabledEnum"=w284) -> ()  [unwired: 2 in, 2 out]
            n179 = property on="Tab Control" class="TabCtl (strict)"("PageSelVis"=w282) -> ()  [unwired: 2 in, 2 out]
            n180 = Read from Text File(file (use dialog)="file path") -> (text=w299:string)  [unwired: 3 in, 3 out]
            n181 = Search and Replace String(replace all?=w293, input string=w299, search string="(", replace string="" ("replace string (\"\")")) -> (result string=w298:string)  [unwired: 4 in, 3 out]
            n182 = Search and Replace String(replace all?=w293, input string=w298, search string=")", replace string="" ("replace string (\"\")")) -> (result string=w300:string)  [unwired: 4 in, 3 out]
            n183 = Search and Replace String(replace all?=w293, input string=w300, search string=",", replace string=" " ("replace string (\"\")")) -> (result string=w306:string)  [unwired: 4 in, 3 out]
            n184 = Search and Replace String(replace all?=w293, input string=w306, search string=".", replace string="," ("replace string (\"\")")) -> (result string=w302:string)  [unwired: 4 in, 3 out]
            n185 = Spreadsheet String To Array(delimiter (Tab)=" ", format string="%f", spreadsheet string=w302) -> (array=w285:dbl[][])  [unwired: 1 in]
            "?" <- w285
            n186 = for {
              N: 14 -> [_]
              tunnel: w285 -> [w350]
              tunnel: [w348] -> w288 mode=indexing
              tunnel: [w347] -> w287 mode=indexing
              tunnel: [w346] -> w286 mode=indexing
              tunnel: [w345] -> w290 mode=indexing
              tunnel: [w344] -> w289 mode=indexing
              i -> [w349]
              n187 = Index Array(array=w350, index (col)=w349) -> (element=w343:dbl[])  [unwired: 1 in]
              n188 = Array Max & Min(array=w343) -> (max value=w345:dbl, min value=w344:dbl)  [unwired: 2 out]
              n189 = call <vilib>:"Std Deviation and Variance.vi"("X"=w343) -> ("mean"=w348:dbl, "standard deviation"=w347:dbl, "variance"=w346:dbl)  [unwired: 1 in]
            }
            "Max 3" <- w290
            "Min 3" <- w289
            "Mean 3" <- w288
            "St. dev 3" <- w287
            "Variance 3" <- w286
            n190 = while {
              tunnel: w285 -> [w314]
              stop <- "stop" stop-if-true
              # "Luce ciclo-->"
              # "applico l'opzione per il filtro"
              n191 = call "one matrix 1-14 graph.vi"("dt"="dt 3", "Applica filtro 4"="Filter 3", "Dati 2"=w314) -> ("Waveform Graph"=→"Waveform Graph":waveform(dbl)[])
              n192 = property on="Waveform Graph" class="WFGraph (strict)"("Active Plot"=u32 0, "Plot.Visible?"="?", "Active Plot"=u32 1, "Plot.Visible?"="?", "Active Plot"=u32 2, "Plot.Visible?"="?", "Active Plot"=u32 3, "Plot.Visible?"="?", "Active Plot"=u32 4, "Plot.Visible?"="?", "Active Plot"=u32 5, "Plot.Visible?"="?", "Active Plot"=u32 6, "Plot.Visible?"="?") -> ()  [unwired: 2 in, 2 out]
              n193 = Not(x="stop") -> (.not. x?=→"Read File":bool)
              n194 = property on="Tab Control" class="TabCtl (strict)"("PageSelVis"="stop") -> ()  [unwired: 2 in, 2 out]
              n195 = property on="Waveform Graph" class="WFGraph (strict)"("Active Plot"=u32 7, "Plot.Visible?"="?", "Active Plot"=u32 8, "Plot.Visible?"="?", "Active Plot"=u32 9, "Plot.Visible?"="?", "Active Plot"=u32 10, "Plot.Visible?"="?", "Active Plot"=u32 11, "Plot.Visible?"="?", "Active Plot"=u32 12, "Plot.Visible?"="?", "Active Plot"=u32 13, "Plot.Visible?"="?") -> ()  [unwired: 2 in, 2 out]
            }
          }
          event "Add": Value Change {
            n196 = event-data() -> ()  [unwired: 1 in, 5 out]
            n197 = Build Array("ID", "PASS") -> (w354:string[])
            n198 = call-poly <vilib>:"Write To Spreadsheet File.vi"("append to file? (new file:F)"=TRUE, "1D data"=w354, "file path (dialog if empty)"=w351) -> ()  [unwired: 5 in, 1 out]
          }
          event "Show": Value Change {
            n199 = event-data() -> ()  [unwired: 1 in, 5 out]
            n200 = call-poly <vilib>:"Read From Spreadsheet File.vi"("file path (dialog if empty)"=w356) -> ("all rows"=→"Username & Password":string[][])  [unwired: 6 in, 4 out]
          }
          event "Delete": Value Change {
            # "Uso while invece che for perchè posso controllare meglio la condizione di fine ciclo"
            # "Il while si ferma se trovo un match nella matrice oppure\n se l'indice i è maggiore della dimensione dell'array"
            # "Cerco index dell'ID da eliminare"
            # "prendo soo gli ID"
            n201 = event-data() -> ()  [unwired: 1 in, 5 out]
            n202 = call-poly <vilib>:"Read From Spreadsheet File.vi"("file path (dialog if empty)"=w358) -> ("all rows"=w368:string[][])  [unwired: 6 in, 4 out]
            n203 = Index Array(array=w368, index (col)=0 ("disabled index (col)")) -> (element=w365:string[])  [unwired: 1 in]
            n204 = Array Size(array=w365) -> (size(s)=w364:i32)
            n205 = while {
              tunnel: w365 -> [w377] mode=indexing
              tunnel: "Delete ID" -> [w376]
              tunnel: [w373] -> w367
              tunnel: w364 -> [w372]
              tunnel: [w371] -> w363
              i -> [w373]
              stop <- w375 stop-if-true
              n206 = Equal?(x=w377, y=w376) -> (x = y?=w371:bool)
              n207 = Greater?(x=w373, y=w372) -> (0:w374:bool)
              n208 = Or(x=w371, y=w374) -> (x .or. y?=w375:bool)
            }
            n209 = Delete From Array(array=w368, length=1, index (row)=w367) -> (array with subset deleted=w359:string[][])  [unwired: 1 in, 1 out]
            n210 = Select(t="Trovato", s=w363, f="Non esiste") -> (s? t:f=→"Result":string)
            n211 = call-poly <vilib>:"Write To Spreadsheet File.vi"("2D data"=w359, "file path (dialog if empty)"=w358) -> ()  [unwired: 6 in, 1 out]
          }
          event "Lock Location": Value Change {
            # "<-- Salvo momentaneamente la scelta in un indicatore"
            # "riferito al tato 13"
            # "disattivo location read file"
            # "disattivo location load file"
            # "se i tasti sono attivi, li disattivo e viceversa\ncontrollo solo il primo tasto perchè poi li tratto insieme"
            # "disattivo location bluetooth"
            n212 = event-data() -> ()  [unwired: 1 in, 5 out]
            n213 = property class="Bool (strict)"() -> ("DisabledEnum"=w411:T2)  [unwired: 2 in, 2 out]
            n214 = local read "Control Option"() -> (w378:string)
            n215 = case shown="\"Enabled\", Default" w411 {
              tunnel: [w421 w425 w428] -> w410
              tunnel: [w421 w425 w428] -> w409
              tunnel: [w421 w425 w428] -> w408
              tunnel: [w422 _ _] -> w393
              tunnel: [w422 _ _] -> w392
              tunnel: [w422 _ _] -> w385
              tunnel: [w421 w425 w428] -> w391
              tunnel: [w422 _ _] -> w390
              tunnel: [w422 FALSE TRUE] -> w384
              tunnel: ["N" "Y" "Y"] -> w382
              frame "Enabled", Default {
                w422 = FALSE
                w421 = 2
              }
              frame "Disabled" {
                w425 = 0
              }
              frame "Disabled and Grayed Out" {
                w428 = 0
              }
            }
            n216 = Replace Substring(2:1 ("length (len. of substring)"), 3:11 ("offset (0)"), 4:w382, 5:w378) -> (1:w379:string)  [unwired: 1 out]
            n217 = local write "Control Option"(w379) -> ()
            n218 = Not(x=w384) -> (.not. x?=→"Stato locat (disabilitato)":bool)
            n219 = property class="Bool (strict)"("DisabledEnum"=w409, "Value"=w392) -> ()  [unwired: 2 in, 2 out]
            n220 = property class="Bool (strict)"("DisabledEnum"=w408, "Value"=w385) -> ()  [unwired: 2 in, 2 out]
            n221 = property class="Bool (strict)"("DisabledEnum"=w410, "Value"=w393) -> ()  [unwired: 2 in, 2 out]
            n222 = property class="Bool (strict)"("DisabledEnum"=w391, "Value"=w390) -> ()  [unwired: 2 in, 2 out]
            n223 = property class="Bool (strict)"() -> ("DisabledEnum"=w407:T2)  [unwired: 2 in, 2 out]
            n224 = case shown="\"Enabled\", Default" w407 {
              tunnel: [w417 w418 w419] -> w406
              tunnel: [w417 w418 w419] -> w405
              tunnel: [w417 w418 w419] -> w404
              tunnel: [w416 _ _] -> w403
              tunnel: [w416 _ _] -> w402
              tunnel: [w416 _ _] -> w401
              tunnel: [w417 w418 w419] -> w389
              tunnel: [w416 _ _] -> w388
              frame "Enabled", Default {
                w416 = FALSE
                w417 = 2
              }
              frame "Disabled" {
                w418 = 0
              }
              frame "Disabled and Grayed Out" {
                w419 = 0
              }
            }
            n225 = property class="Bool (strict)"("DisabledEnum"=w389, "Value"=w388) -> ()  [unwired: 2 in, 2 out]
            n226 = property class="Bool (strict)"("DisabledEnum"=w406, "Value"=w403) -> ()  [unwired: 2 in, 2 out]
            n227 = property class="Bool (strict)"("DisabledEnum"=w405, "Value"=w402) -> ()  [unwired: 2 in, 2 out]
            n228 = property class="Bool (strict)"("DisabledEnum"=w404, "Value"=w401) -> ()  [unwired: 2 in, 2 out]
            n229 = property class="Bool (strict)"() -> ("DisabledEnum"=w400:T2)  [unwired: 2 in, 2 out]
            n230 = case shown="\"Disabled\"" w400 {
              tunnel: [w413 w414 w415] -> w399
              tunnel: [w413 w414 w415] -> w398
              tunnel: [w413 w414 w415] -> w397
              tunnel: [w412 _ _] -> w394
              tunnel: [w412 _ _] -> w395
              tunnel: [w412 _ _] -> w396
              tunnel: [w413 w414 w415] -> w387
              tunnel: [w412 _ _] -> w386
              frame "Enabled", Default {
                w412 = FALSE
                w413 = 2
              }
              frame "Disabled" {
                w414 = 0
              }
              frame "Disabled and Grayed Out" {
                w415 = 0
              }
            }
            n231 = property class="Bool (strict)"("DisabledEnum"=w387, "Value"=w386) -> ()  [unwired: 2 in, 2 out]
            n232 = property class="Bool (strict)"("DisabledEnum"=w399, "Value"=w394) -> ()  [unwired: 2 in, 2 out]
            n233 = property class="Bool (strict)"("DisabledEnum"=w398, "Value"=w395) -> ()  [unwired: 2 in, 2 out]
            n234 = property class="Bool (strict)"("DisabledEnum"=w397, "Value"=w396) -> ()  [unwired: 2 in, 2 out]
          }
          event "Lock Distance": Value Change {
            # "Dissattivo/riattivo il tastino della distanza.\nSe lo disattivo setto anche il suo valore su False"
            # "Read file"
            # "Load file"
            # "Bluetooth"
            # "Riferito al 9 tastino bluetooth"
            n235 = event-data() -> ()  [unwired: 1 in, 5 out]
            n236 = local read "Control Option"() -> (w431:string)
            n237 = property class="Bool (strict)"() -> ("DisabledEnum"=w438:T2)  [unwired: 2 in, 2 out]
            n238 = case shown="\"Disabled and Grayed Out\"" w438 {
              tunnel: [2 0 0] -> w437
              tunnel: [w440 _ _] -> w436
              tunnel: [w440 FALSE TRUE] -> w435
              tunnel: ["N" "Y" "Y"] -> w429
              frame "Enabled", Default {
                w440 = FALSE
              }
              frame "Disabled" {
              }
              frame "Disabled and Grayed Out" {
              }
            }
            n239 = Replace Substring(2:1 ("length (len. of substring)"), 3:25 ("offset (0)"), 4:w429, 5:w431) -> (1:w430:string)  [unwired: 1 out]
            n240 = local write "Control Option"(w430) -> ()
            n241 = Not(x=w435) -> (.not. x?=→"Stato DIst (disabilitato)":bool)
            n242 = property class="Bool (strict)"("DisabledEnum"=w437, "Value"=w436) -> ()  [unwired: 2 in, 2 out]
            n243 = property class="Bool (strict)"("DisabledEnum"=w437, "Value"=w436) -> ()  [unwired: 2 in, 2 out]
            n244 = property class="Bool (strict)"("DisabledEnum"=w437, "Value"=w436) -> ()  [unwired: 2 in, 2 out]
          }
          event "QUIT": Value Change {
            # "Salvo in un file txt la scelta dell'admin \nsu Lock location/distance"
            # "Disabilito la Tab alla chiusura del programma"
            n245 = event-data() -> ()  [unwired: 1 in, 5 out]
            n246 = call <vilib>:"Application Directory.vi"() -> ("Application Directory"=w450:path)
            n247 = Build Path(base path=w450, name or relative path="Option_Control.txt") -> (appended path=w448:path)
            n248 = local read "Control Option"() -> (w451:string)
            n249 = Boolean To (0,1)(Boolean="QUIT") -> (0, 1=w455:i16)
            n250 = Multiply(x=w455, y=i16 2) -> (x*y=w454:i16)
            n251 = Write to Text File(file (use dialog)=w448, text=w451) -> ()  [unwired: 2 in, 3 out]
            n252 = property on="Tab Control" class="TabCtl (strict)"("DisabledEnum"=w454) -> ()  [unwired: 2 in, 2 out]
          }
        }
      }
    }
  }
  n253 = control-ref of="This VI"() -> (w1:refnum<vi>)
  n254 = invoke class="VI" method="Default Vals.Reinit All"(reference=w1) -> ()  [unwired: 2 in, 3 out]
